vi "Detector_COM.vi"(8 "error in (no error)":errorcluster, 10 "Selector":string(combo)) -> (0 "error out":errorcluster, 2 "find list":string[](array[string]))   [LabVIEW 2025]
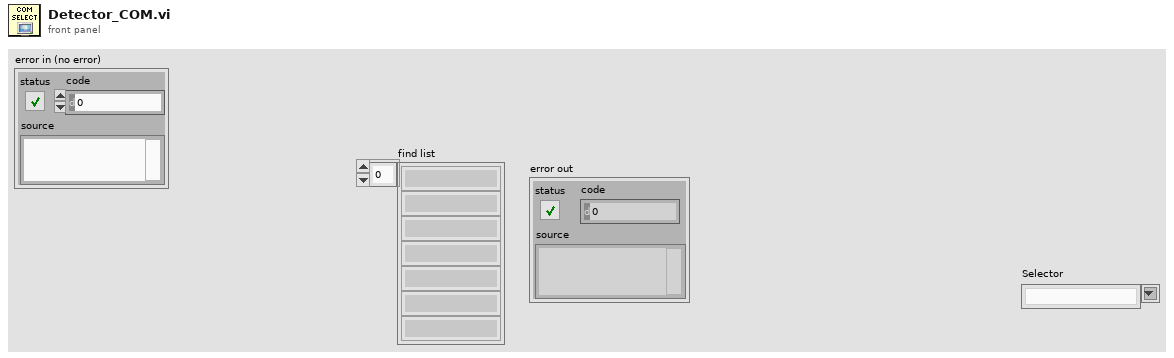
[diagram p1: front panel]
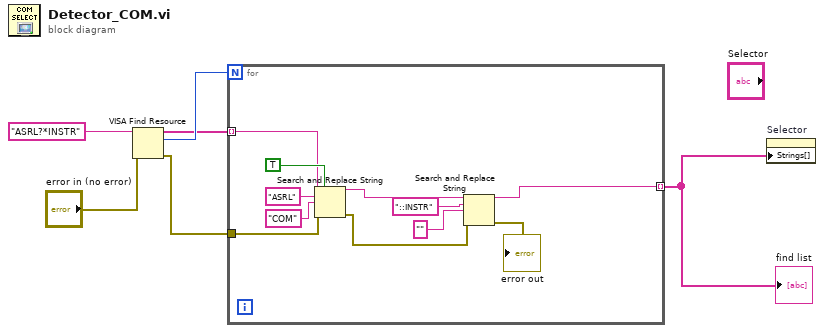
[diagram p0: block diagram]
diagram:
  n1 = VISA Find Resource(8:"error in (no error)", 11:"ASRL?*INSTR" ("expression (\"?*\")")) -> (0:w3:errorcluster, 2:w5:u32, 3:w4:string[])  [unwired: 1 in]
  n2 = for {
    N: w5 -> [_]
    tunnel: w4 -> [w14] mode=indexing
    tunnel: w3 -> [w10]
    tunnel: [w7] -> w1 mode=indexing
    n3 = Search and Replace String(replace all?=TRUE ("replace all? (F)"), input string=w14, search string="ASRL", replace string="COM" ("replace string (\"\")"), error in=w10) -> (result string=w13:string, error out=w9:errorcluster)  [unwired: 3 in, 2 out]
    n4 = Search and Replace String(input string=w13, search string="::INSTR", replace string="" ("replace string (\"\")"), error in=w9) -> (result string=w7:string, error out=→"error out":errorcluster)  [unwired: 4 in, 2 out]
  }
  "find list" <- w1
  n5 = property on="Selector" class="CmbBox"("Strings[]"=w1) -> ()  [unwired: 2 in, 2 out]
